vi "Check for Cluster.vi"(8 "error in (no error)":errorcluster, 11 "TDMS in":refnum<class "TDMS.lvclass">) -> (0 "error out":errorcluster, 3 "TDMS out":refnum<class "TDMS.lvclass">)   [LabVIEW 2019, in "TDMS.lvlib" / "TDMS.lvclass"]
uses:
  TDMS.lvclass
  TDMS.lvclass/TDMS.ctl
  <vilib>/Utility/Data Type/NI_Data Type.lvlib
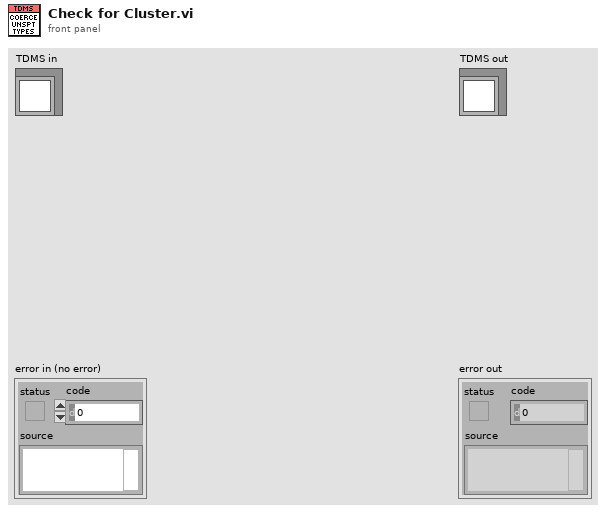
[diagram p1: front panel]
types:
  T1 = typedef "NI_Data Type.lvlib/Data Type.ctl" = enum8{"Invalid Type", "Void", "I8", "I16", "I32", "I64", "U8", "U16", "U32", "U64", "Single Float", "Double Float", "Extended Float", "Single Complex", "Double Complex", "Extended Complex", "Enum U8", "Enum U16", "Enum U32", "Enum U64", "Single Float With Unit", "Double Float With Unit", "Extended Float With Unit", "Single Complex with Unit", "Double Complex with Unit", "Extended Complex with Unit", "Boolean", "String", "Path", "Picture", "Tag", "Array", "Cluster", "Variant", "LV Variant", "Waveform", "Timestamp", "Digital Waveform", "Digital Data", "ExpressData", "Refnum", "External Data", "VI", "Poly VI", "LabVIEW Class Instance", "Fixed Point", "Set Collection", "Map Collection"}
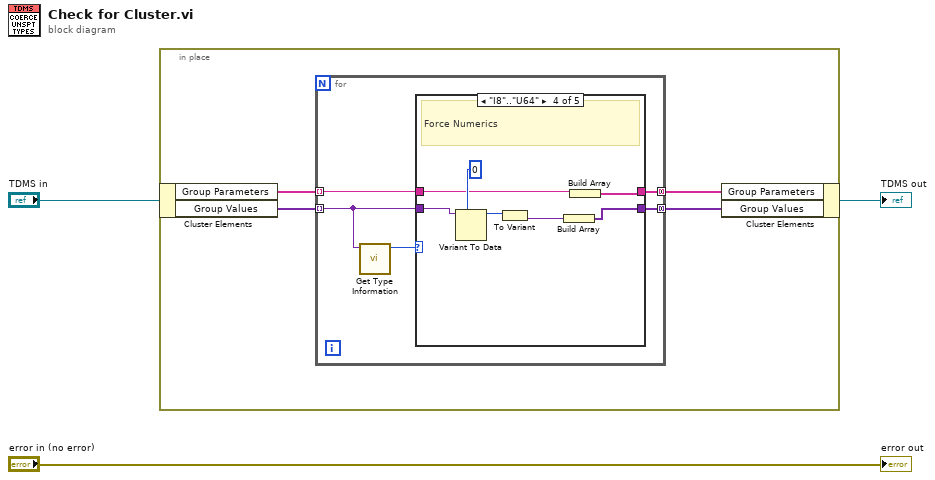
[diagram p0: block diagram]
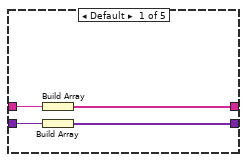
[diagram p2: hidden frame]
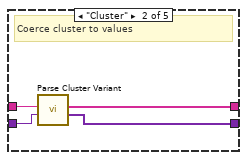
[diagram p3: hidden frame]
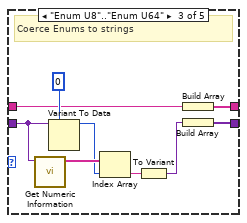
[diagram p4: hidden frame]
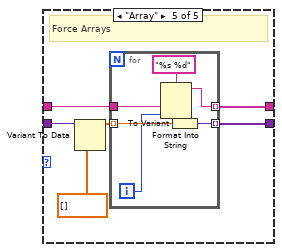
[diagram p5: hidden frame]
diagram:
  n1 = in-place {
    n2 = in-place-cluster #1("TDMS in") -> ("Group Parameters"=w7:string[], "Group Values"=w6:variant[])
    n3 = for {
      tunnel: w7 -> [w11] mode=indexing
      tunnel: w6 -> [w9] mode=indexing
      tunnel: [w10] -> w5 mode=concatenating
      tunnel: [w8] -> w4 mode=concatenating
      n4 = call <vilib>:"Get Type Information.vi"("variant"=w9) -> ("type"=w12:T1)  [unwired: 6 in, 4 out]
      n5 = case shown="\"I8\"..\"U64\"" w12 {
        tunnel: w11 -> [w16 w20 w25 w33 w38]
        tunnel: [w15 w19 w24 w32 w37] -> w10
        tunnel: w9 -> [w14 w18 w28 w36 w42]
        tunnel: [w13 w17 w21 w30 w39] -> w8
        frame Default {
          n6 = Build Array(w16) -> (w15:string[])
          n7 = Build Array(w14) -> (w13:variant[])
        }
        frame "Cluster" {
          # "Coerce cluster to values"
          n8 = call "Parse Cluster Variant.vi"("Cluster Variant in"=w18, "Group Parameters in"=w20) -> ("appended array"=w17:variant[], "Group Parameters out"=w19:string[])  [unwired: 8 in]
        }
        frame "Enum U8".."Enum U64" {
          # "Coerce Enums to strings"
          n9 = call <vilib>:"Get Numeric Information.vi"("variant"=w28) -> ("enum names"=w29:string[])  [unwired: 7 in, 3 out]
          n10 = Variant To Data(type=i64 0, Variant=w28) -> (data=w27:i64)  [unwired: 1 in, 1 out]
          n11 = Index Array(array=w29, index=w27) -> (element=w23:string)
          n12 = To Variant(anything=w23) -> (Variant=w22:variant)
          n13 = Build Array(w25) -> (w24:string[])
          n14 = Build Array(w22) -> (w21:variant[])
        }
        frame "I8".."U64" {
          # "Force Numerics"
          n15 = Variant To Data(type=i64 0, Variant=w36) -> (data=w34:i64)  [unwired: 1 in, 1 out]
          n16 = To Variant(anything=w34) -> (Variant=w31:variant)
          n17 = Build Array(w31) -> (w30:variant[])
          n18 = Build Array(w33) -> (w32:string[])
        }
        frame "Array" {
          # "Force Arrays"
          n19 = Variant To Data(type=dbl[] [], Variant=w42) -> (data=w40:dbl[])  [unwired: 1 in, 1 out]
          n20 = for {
            tunnel: w40 -> [w48] mode=indexing
            tunnel: [w47] -> w39 mode=indexing
            tunnel: w38 -> [w45]
            tunnel: [w43] -> w37 mode=indexing
            i -> [w44]
            n21 = Format Into String(format string="%s %d", w45, w44) -> (resulting string=w43:string)  [unwired: 2 in, 1 out]
            n22 = To Variant(anything=w48) -> (Variant=w47:variant)
          }
        }
      }
    }
    n23 = in-place-cluster #1("Group Parameters"=w5, "Group Values"=w4) -> (→"TDMS out":refnum<class "TDMS.lvclass">)
  }
  "error out" <- "error in (no error)"
